vi "Memory.Pointer.Bounds Check.Size.vi"(8 "error in (no error)":errorcluster, 10 "size":i64 format="%d bytes", 11 "Pointer in":refnum<class "Memory.Pointer.lvclass">) -> (0 "error out":errorcluster, 1 "size valid":bool, 2 "size out":i64 format="%d bytes", 3 "Pointer out":refnum<class "Memory.Pointer.lvclass">)   [LabVIEW 2016, in "LabVIEW Memory Manager.lvlib" / "Memory.Pointer.lvclass"]
uses:
  Memory.Pointer.lvclass
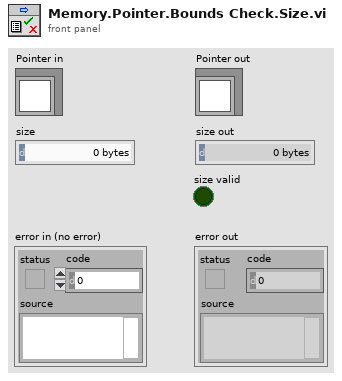
[diagram p1: front panel]
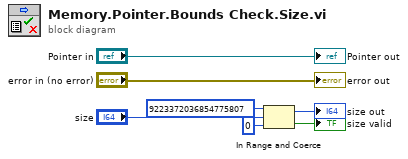
[diagram p0: block diagram]
diagram:
  n1 = In Range and Coerce(upper limit=i64 9223372036854775807, x="size", lower limit=i64 0) -> (coerced(x)=→"size out":i64, In Range?=→"size valid":bool)
  "error out" <- "error in (no error)"
  "Pointer out" <- "Pointer in"
